vi "test_libssh2_channel_handle_extended_data2.vi"(8 "stderr":string, 9 "stdout":string, 10 "stdin":string, 11 "mode":i32) -> (0 "error out":errorcluster)   [LabVIEW 2017, in "integration_tests.lvlib"]
uses:
  integration_tests.lvlib
  libssh2/libssh2_channel_open_ex.vi
  libssh2/libssh2_channel_process_startup.vi
  libssh2/libssh2_channel_read_ex.vi
  support/support.lvlib
  libssh2/libssh2.lvlib
  <vilib>/PNR/Transparent Assertions/Transparent Assertions/Transparent Assertions.lvlib
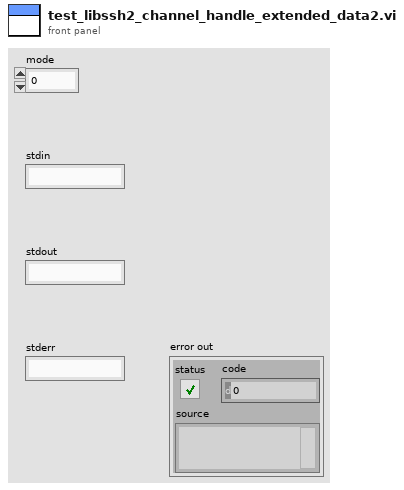
[diagram p1: front panel]
types:
  T1 = typedef "libssh2.lvlib/Session Refnum.ctl" = refnum<k1>
  T2 = typedef "libssh2.lvlib/Channel Refnum.ctl" = refnum<k1>
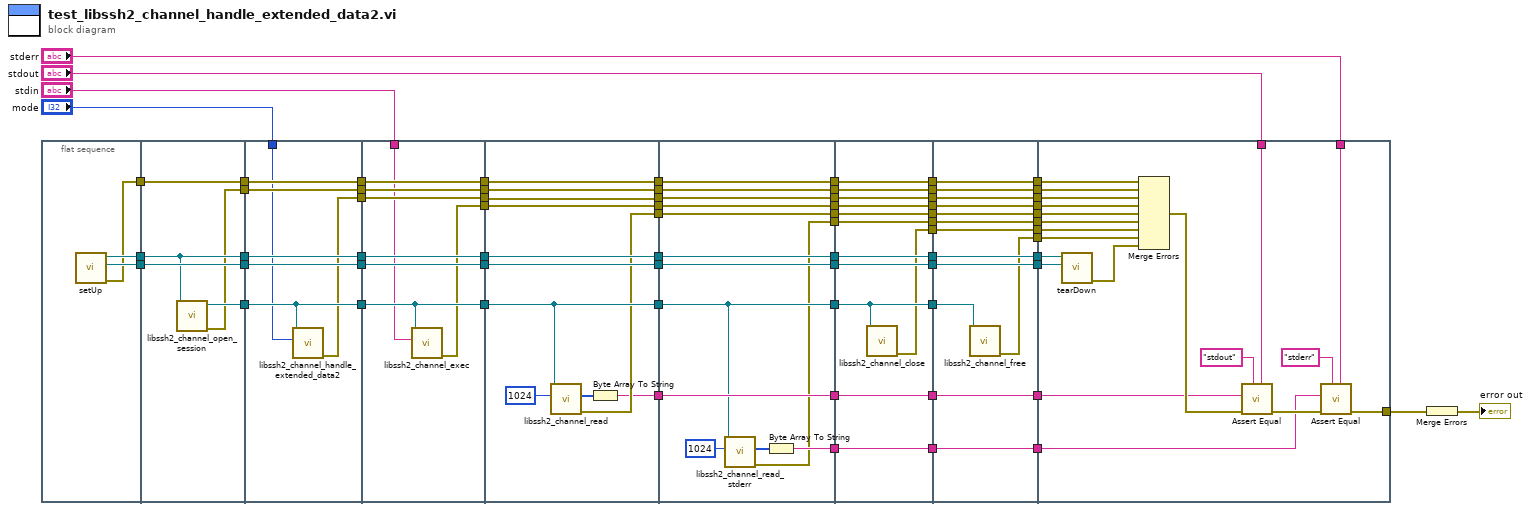
[diagram p0: block diagram]
diagram:
  n1 = flat-sequence {
    tunnel: [w74] -> w65
    tunnel: [w73] -> w64
    tunnel: [w72] -> w63
    tunnel: w65 -> [w78]
    tunnel: w64 -> [w79]
    tunnel: [w78] -> w62
    tunnel: [w79] -> w61
    tunnel: [w77] -> w60
    tunnel: w63 -> [w76]
    tunnel: [w76] -> w59
    tunnel: [w75] -> w58
    tunnel: w62 -> [w86]
    tunnel: [w86] -> w57
    tunnel: w61 -> [w85]
    tunnel: [w85] -> w56
    tunnel: w60 -> [w82]
    tunnel: [w82] -> w55
    tunnel: w59 -> [w84]
    tunnel: [w84] -> w54
    tunnel: w58 -> [w83]
    tunnel: [w83] -> w53
    tunnel: "mode" -> [w81]
    tunnel: [w80] -> w52
    tunnel: w57 -> [w94]
    tunnel: [w94] -> w51
    tunnel: w56 -> [w93]
    tunnel: [w93] -> w50
    tunnel: w55 -> [w91]
    tunnel: [w91] -> w49
    tunnel: w54 -> [w92]
    tunnel: [w92] -> w48
    tunnel: w53 -> [w90]
    tunnel: [w90] -> w47
    tunnel: [w89] -> w46
    tunnel: w52 -> [w88]
    tunnel: [w88] -> w45
    tunnel: "stdin" -> [w87]
    tunnel: w51 -> [w105]
    tunnel: [w105] -> w44
    tunnel: w50 -> [w104]
    tunnel: [w104] -> w43
    tunnel: w49 -> [w98]
    tunnel: [w98] -> w42
    tunnel: w48 -> [w103]
    tunnel: [w103] -> w41
    tunnel: w47 -> [w102]
    tunnel: [w102] -> w40
    tunnel: w46 -> [w101]
    tunnel: [w101] -> w39
    tunnel: [w97] -> w38
    tunnel: w45 -> [w100]
    tunnel: [w100] -> w37
    tunnel: [w95] -> w36
    tunnel: w44 -> [w118]
    tunnel: [w118] -> w35
    tunnel: w43 -> [w117]
    tunnel: [w117] -> w34
    tunnel: w42 -> [w110]
    tunnel: [w110] -> w33
    tunnel: w41 -> [w116]
    tunnel: [w116] -> w32
    tunnel: w40 -> [w115]
    tunnel: [w115] -> w31
    tunnel: w39 -> [w114]
    tunnel: [w114] -> w30
    tunnel: w38 -> [w113]
    tunnel: [w113] -> w29
    tunnel: w37 -> [w112]
    tunnel: [w112] -> w28
    tunnel: w36 -> [w111]
    tunnel: [w111] -> w27
    tunnel: [w107] -> w26
    tunnel: [w106] -> w25
    tunnel: w35 -> [w130]
    tunnel: w34 -> [w129]
    tunnel: w33 -> [w128]
    tunnel: [w130] -> w24
    tunnel: [w129] -> w23
    tunnel: [w128] -> w22
    tunnel: [w127] -> w21
    tunnel: w32 -> [w126]
    tunnel: [w126] -> w20
    tunnel: w31 -> [w125]
    tunnel: [w125] -> w19
    tunnel: w30 -> [w124]
    tunnel: [w124] -> w18
    tunnel: w29 -> [w123]
    tunnel: [w123] -> w17
    tunnel: w28 -> [w122]
    tunnel: [w122] -> w15
    tunnel: [w121] -> w16
    tunnel: w27 -> [w121]
    tunnel: [w120] -> w14
    tunnel: w26 -> [w120]
    tunnel: w25 -> [w119]
    tunnel: [w119] -> w13
    tunnel: w24 -> [w143]
    tunnel: w23 -> [w142]
    tunnel: w22 -> [w141]
    tunnel: [w143] -> w12
    tunnel: [w142] -> w11
    tunnel: [w140] -> w10
    tunnel: w21 -> [w139]
    tunnel: [w139] -> w9
    tunnel: w20 -> [w138]
    tunnel: [w138] -> w8
    tunnel: w19 -> [w137]
    tunnel: [w137] -> w7
    tunnel: w18 -> [w136]
    tunnel: [w136] -> w6
    tunnel: w17 -> [w135]
    tunnel: [w135] -> w5
    tunnel: [w134] -> w4
    tunnel: w16 -> [w134]
    tunnel: w15 -> [w133]
    tunnel: [w133] -> w3
    tunnel: [w132] -> w2
    tunnel: w14 -> [w132]
    tunnel: w13 -> [w131]
    tunnel: [w131] -> w1
    tunnel: w12 -> [w163]
    tunnel: w11 -> [w162]
    tunnel: [w147] -> w71
    tunnel: w10 -> [w160]
    tunnel: w9 -> [w159]
    tunnel: w8 -> [w158]
    tunnel: w7 -> [w156]
    tunnel: w6 -> [w155]
    tunnel: w5 -> [w154]
    tunnel: w4 -> [w153]
    tunnel: w3 -> [w152]
    tunnel: "stdout" -> [w151]
    tunnel: w2 -> [w144]
    tunnel: w1 -> [w149]
    tunnel: "stderr" -> [w145]
    frame #0 {
      n2 = call "setUp.vi"() -> ("error out"=w72:errorcluster, "connection ID"=w73:refnum<k5>, "session"=w74:T1)  [unwired: 9 in]
    }
    frame #1 {
      n3 = call "libssh2_channel_open_session.vi"("session"=w78) -> ("error out"=w75:errorcluster, "channel"=w77:T2)  [unwired: 9 in]
    }
    frame #2 {
      n4 = call "libssh2_channel_handle_extended_data2.vi"("mode (normal)"=w81, "channel"=w82) -> ("error out"=w80:errorcluster)  [unwired: 9 in]
    }
    frame #3 {
      n5 = call "libssh2_channel_exec.vi"("command"=w87, "channel"=w91) -> ("error out"=w89:errorcluster)  [unwired: 9 in]
    }
    frame #4 {
      n6 = call "libssh2_channel_read.vi"("buffer length"=1024, "channel"=w98) -> ("error out"=w97:errorcluster, "buffer"=w96:u8[])  [unwired: 8 in]
      n7 = Byte Array To String(unsigned byte array=w96) -> (string=w95:string)
    }
    frame #5 {
      n8 = call "libssh2_channel_read_stderr.vi"("buffer length"=1024, "channel"=w110) -> ("error out"=w106:errorcluster, "buffer"=w108:u8[])  [unwired: 8 in]
      n9 = Byte Array To String(unsigned byte array=w108) -> (string=w107:string)
    }
    frame #6 {
      n10 = call "libssh2_channel_close.vi"("channel"=w128) -> ("error out"=w127:errorcluster)  [unwired: 10 in]
    }
    frame #7 {
      n11 = call "libssh2_channel_free.vi"("channel"=w141) -> ("error out"=w140:errorcluster)  [unwired: 10 in]
    }
    frame #8 {
      n12 = call "tearDown.vi"("connection ID"=w162, "session"=w163) -> ("error out"=w161:errorcluster)  [unwired: 9 in]
      n13 = Merge Errors(w158, w156, w152, w155, w154, w149, w159, w160, w161) -> (w157:errorcluster)
      n14 = call <vilib>:"Assert Equal.vi"("Expected"=w151, "Message (\"\")"="stdout" ("Label"), "error in (no error)"=w157, "Actual"=w153) -> ("error out"=w148:errorcluster)  [unwired: 7 in]
      n15 = call <vilib>:"Assert Equal.vi"("Expected"=w145, "Message (\"\")"="stderr" ("Label"), "error in (no error)"=w148, "Actual"=w144) -> ("error out"=w147:errorcluster)  [unwired: 7 in]
    }
  }
  n16 = Merge Errors(w71) -> (→"error out":errorcluster)
